vi "PriorityQueue Usage Example1.vi"() -> ()   [LabVIEW 2009]
doc: "This example demonstrates the basic sorting capabilities of a priority queue."
uses:
  PriorityQueue/PriorityQueue.lvclass
panel:
  in  "Enqueued Elements":cluster{"Element":string, "Priority":i32}[](array[cluster])=[{"Element"="c", "Priority"=2}, {"Element"="e", "Priority"=4}, {"Element"="b", "Priority"=1}, {"Element"="z", "Priority"=-1}, {"Element"="d", "Priority"=3}, {"Element"="a", "Priority"=0}, {"Element"="oops", "Priority"=2}]
  out "error out":errorcluster
  out "Dequeued Elements":string[](array[string])
  # "This example creates a priority queue with 5 priority levels, 0-4.  All the elements are added to the queue before any of them are dequeued.  Note that when dequeued the elements are in order according to the priority levels they have been given.\n\nGiving an element a priority level that does not exist (such as -1) results in the element being given the lowest possible priority (4 in this case) and added to the queue."
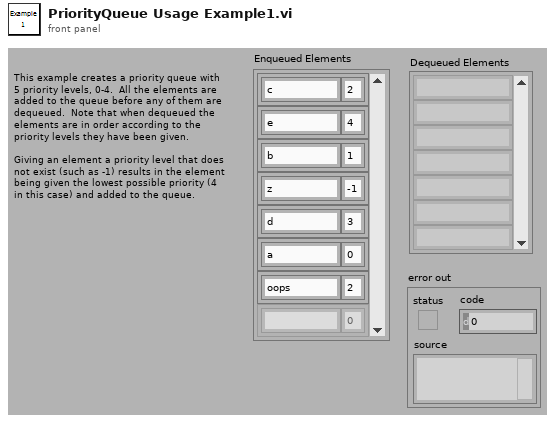
[diagram p1: front panel]
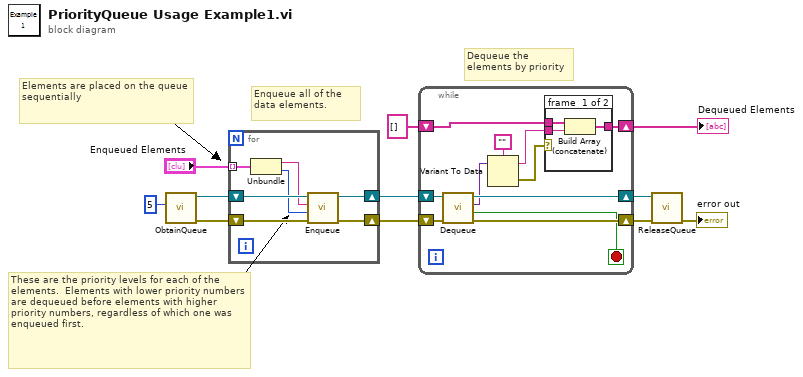
[diagram p0: block diagram]
diagram:
  # "These are the priority levels for each of the elements.  Elements with lower priority numbers are dequeued before elements with higher priority numbers, regardless of which one was enqueued first."
  # "Dequeue the elements by priority"
  # "Enqueue all of the data elements."
  # "Elements are placed on the queue sequentially"
  n1 = call "ObtainQueue.vi"("# Priority Levels (5)"=5) -> ("error out"=w9:errorcluster, "PriorityQueue out"=w10:refnum<class "PriorityQueue.lvclass">)  [unwired: 9 in]
  n2 = for {
    shift-right: [w17] -> w8
    shift-left: w10 -> [w18]
    shift-right: [w15] -> w7
    shift-left: w9 -> [w16]
    tunnel: "Enqueued Elements" -> [w14] mode=indexing
    n3 = Unbundle(w14) -> ("Element"=w12:string, "Priority"=w13:i32)
    n4 = call-dynamic "Enqueue.vi"("error in (no error)"=w16, "Priority Number"=w13, "Element"=w12, "PriorityQueue in"=w18) -> ("error out"=w15:errorcluster, "PriorityQueue out"=w17:refnum<class "PriorityQueue.lvclass">)  [unwired: 6 in]
  }
  n5 = while {
    shift-right: [w27] -> w6
    shift-left: w8 -> [w29]
    shift-right: [w26] -> w5
    shift-left: w7 -> [w28]
    shift-right: [w21] -> w4
    shift-left: string[] [] -> [w20]
    stop <- w25 stop-if-true
    n6 = call-dynamic "Dequeue.vi"("error in (no error)"=w28, "PriorityQueue in"=w29) -> ("error out"=w26:errorcluster, "Timed Out?"=w25:bool, "Element"=w24:variant, "PriorityQueue out"=w27:refnum<class "PriorityQueue.lvclass">)  [unwired: 6 in]
    n7 = Variant To Data(Variant=w24, type="") -> (error out=w19:errorcluster, data=w22:string)  [unwired: 1 in]
    n8 = case shown="No Error" w19 {
      tunnel: w22 -> [w32 _]
      tunnel: [w31 w33] -> w21
      tunnel: w20 -> [w30 w33]
      frame #0 {
        n9 = Build Array (concatenate)(w30, w32) -> (w31:string[])
      }
      frame #1 {
      }
    }
  }
  "Dequeued Elements" <- w4
  n10 = call-dynamic "ReleaseQueue.vi"("error in (no error)"=w5, "PriorityQueue in"=w6) -> ("error out"=→"error out":errorcluster)  [unwired: 9 in]
